vi "AutoPilotTest.vi"() -> ()   [LabVIEW 2018]
panel:
  out "x offset":dbl
  out "theta":dbl
  in  "apparent target width (p)":dbl=10.0 format="%#_13g"
  in  "apparent target height (p)":dbl=10.0 format="%#_13g"
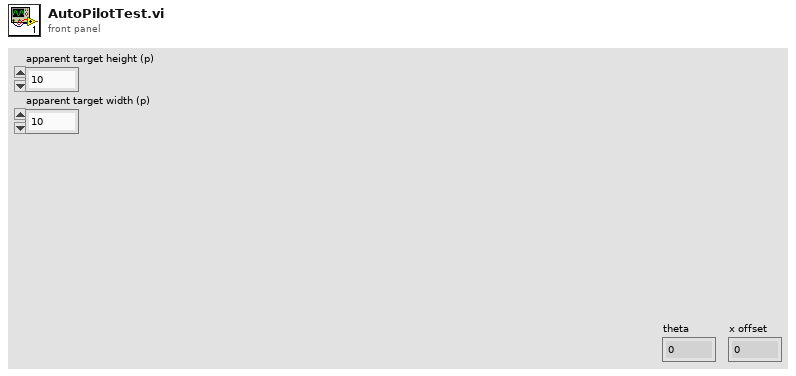
[diagram p1: front panel]
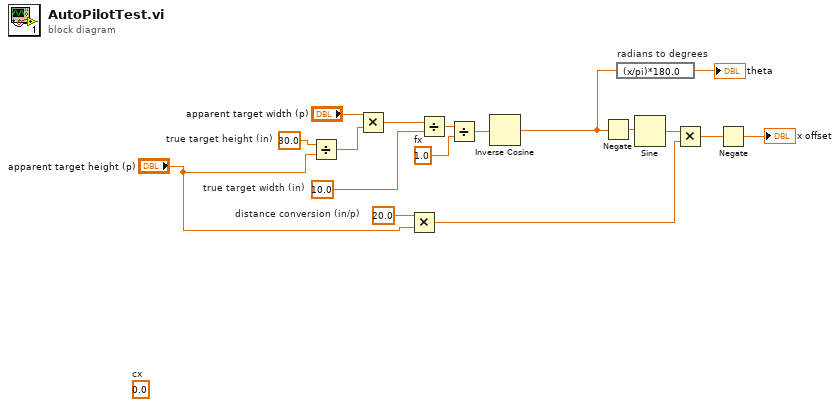
[diagram p0: block diagram]
diagram:
  w8 = 20.0  # distance conversion (in/p)
  w17 = 30.0  # true target height (in)
  w13 = 10.0  # true target width (in)
  (unwired) 0.0  # cx
  w11 = 1.0  # fx
  n1 = Divide(x=w17, y="apparent target height (p)") -> (x/y=w15:dbl)
  n2 = Multiply(x="apparent target width (p)", y=w15) -> (x*y=w14:dbl)
  n3 = Multiply(x=w8, y="apparent target height (p)") -> (x*y=w5:dbl)
  n4 = Divide(x=w14, y=w13) -> (x/y=w12:dbl)
  n5 = Divide(x=w12, y=w11) -> (x/y=w10:dbl)
  n6 = Inverse Cosine(1:w10) -> (0:w2:dbl)
  n7 = Negate(x=w2) -> (-x=w9:dbl)
  n8 = expression code="(x/pi)*180.0" "radians to degrees"(w2) -> (→"theta":dbl)
  n9 = Sine(x=w9) -> (sin(x)=w6:dbl)
  n10 = Multiply(x=w6, y=w5) -> (x*y=w4:dbl)
  n11 = Negate(x=w4) -> (-x=→"x offset":dbl)
